vi "Interepter.vi"(11 "Array":string[][](array[string])) -> ()   [LabVIEW 2011]
uses:
  <vilib>/regexp/Match Regular Expression.xnode
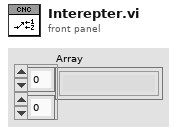
[diagram p1: front panel]
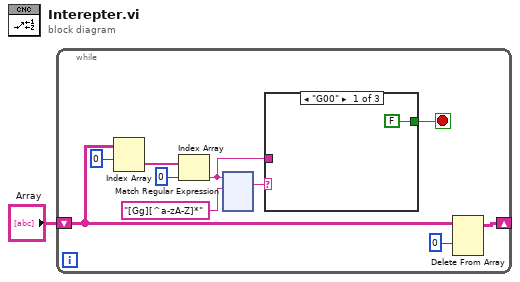
[diagram p0: block diagram]
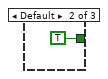
[diagram p2: hidden frame]
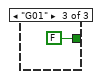
[diagram p3: hidden frame]
diagram:
  n1 = while {
    shift-right: [w10] -> _
    shift-left: "Array" -> [w7]
    stop <- w8 stop-if-true
    n2 = Index Array(array=w7, index (row)=0) -> (element=w6:string[])  [unwired: 1 in]
    n3 = Index Array(array=w6, index=0 ("index (row)")) -> (element=w2:string)
    n4 = xnode "Match Regular Expression"("input string"=w2, "regular expression"="[Gg][^a-zA-Z]*") -> ("whole match"=w3:string)  [unwired: 4 in, 4 out]
    n5 = case shown="\"G00\"" w3 {
      tunnel: [FALSE TRUE FALSE] -> w8
      tunnel: w2 -> [_ _ _]
      frame "G00" {
      }
      frame Default {
      }
      frame "G01" {
      }
    }
    n6 = Delete From Array(array=w7, index (row)=0) -> (array with subset deleted=w10:string[][])  [unwired: 2 in, 1 out]
  }
